vi "Read device.vi"(8 "error in (no error)":errorcluster, 11 "Update Ctl Device Setpoint MSG in":refnum<class "Update Ctl Device Setpoint MSG.lvclass">) -> (0 "error out":errorcluster, 2 "device":string, 3 "Update Ctl Device Setpoint MSG out":refnum<class "Update Ctl Device Setpoint MSG.lvclass">)   [LabVIEW 2016, in "Controller.lvlib" / "Update Ctl Device Setpoint MSG.lvclass"]
uses:
  Update Ctl Device Setpoint MSG.lvclass
  Update Ctl Device Setpoint MSG.lvclass/Update Ctl Device Setpoint MSG.ctl
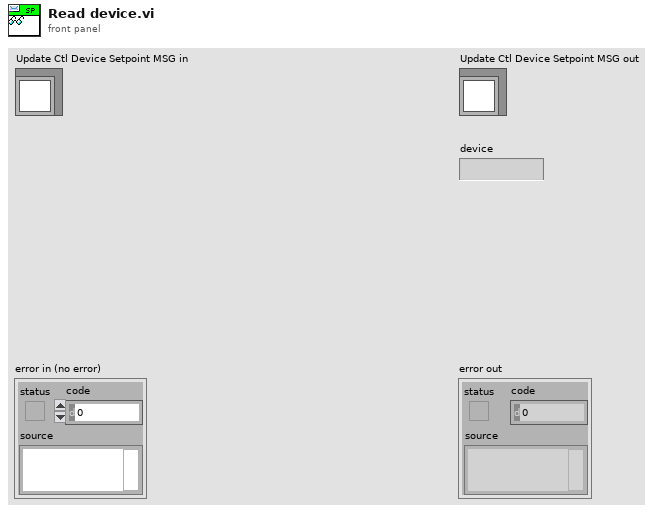
[diagram p1: front panel]
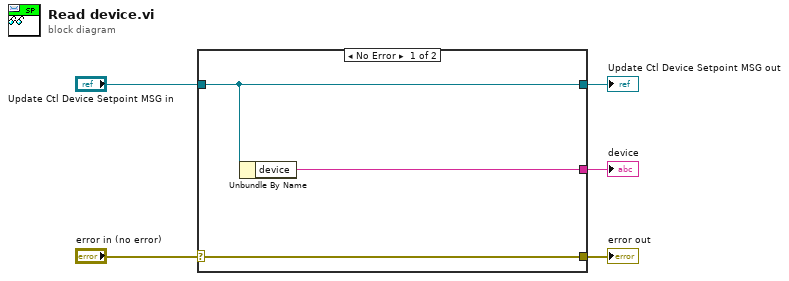
[diagram p0: block diagram]
diagram:
  n1 = case shown="No Error" "error in (no error)" {
    selector: "error in (no error)" -> [w8 w9]
    tunnel: [w8 w9] -> w4
    tunnel: [w7 w10] -> w2
    tunnel: "Update Ctl Device Setpoint MSG in" -> [w7 w10]
    tunnel: [w6 _] -> w1
    frame No Error {
      n2 = Unbundle By Name(w7) -> ("device"=w6:string)
    }
    frame Error {
    }
  }
  "error out" <- w4
  "Update Ctl Device Setpoint MSG out" <- w2
  "device" <- w1
